vi "Camera Manual Control.vi"() -> ()   [LabVIEW 2017]
uses:
  Shared Components/Gantry Class/Gantry Class.lvclass
  Shared Components/Config Manager Class/Type Definitions/Camera Enum.ctl
panel:
  in  "Enable Crosshairs":bool
  out "error out":errorcluster
  in  "stop":bool
  in  "Camera Name":T1
  out "Preview":T2(plugin-control)
  in  "Virtual Mode":bool
  in  "Config Folder":path=path "C:/Users/husker/Desktop/gantry/Config"
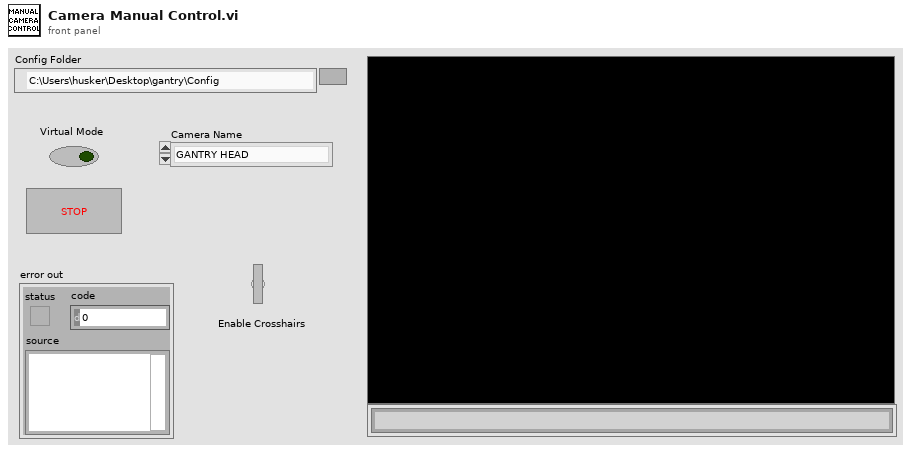
[diagram p1: front panel]
types:
  T1 = typedef "Camera Enum.ctl" = enum16{"GANTRY HEAD", "NEEDLE CALIBRATION X", "NEEDLE CALIBRATION Y", "STAND CAMERA"}
  T2 = typedef "IMAQ Image.ctl" = refnum<image>
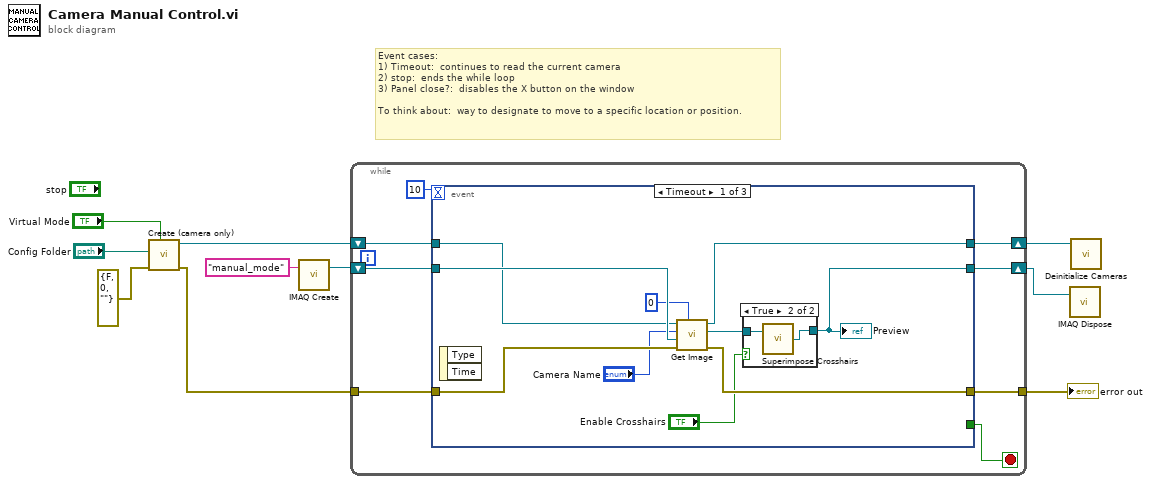
[diagram p0: block diagram]
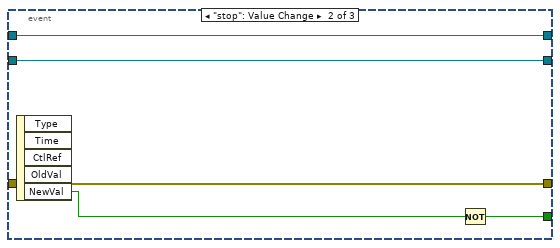
[diagram p3: hidden frame]
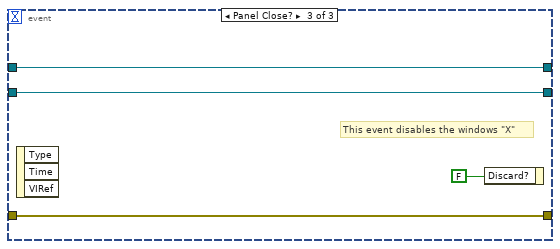
[diagram p4: hidden frame]
diagram:
  # "Event cases:\n1) Timeout:  continues to read the current camera\n2) stop:  ends the while loop\n3) Panel close?:  disables the X button on the window\n\nTo think about:  way to designate to move to a specific location or position."
  n1 = call "Create (camera only).vi"("Virtual Mode"="Virtual Mode", "error in"=errorcluster {"status"=FALSE, "code"=0, "source"=""}, "Config Folder"="Config Folder") -> ("error out"=w4:errorcluster, "Gantry out"=w7:refnum<class "Gantry Class.lvclass">)  [unwired: 7 in]
  n2 = call "IMAQ Create"("Image Name"="manual_mode") -> ("New Image"=w6:T2)  [unwired: 4 in, 1 out]
  n3 = while {
    tunnel: w4 -> [w16]
    tunnel: [w17] -> w2
    shift-right: [w12] -> w1
    shift-left: w6 -> [w13]
    shift-right: [w14] -> w3
    shift-left: w7 -> [w15]
    stop <- w11 stop-if-true
    n4 = event shown="[0] Timeout" {
      selector: _ -> [_ _ _]
      dyn-events: _ -> [_ _ _]
      timeout: 10 -> [_ _ _]
      tunnel: [_ w32 _] -> w11
      tunnel: [w26 w36 w39] -> w17
      tunnel: w16 -> [w23 w36 w39]
      tunnel: w15 -> [w24 w35 w38]
      tunnel: [w28 w35 w38] -> w14
      tunnel: w13 -> [w27 w34 w37]
      tunnel: [w20 w34 w37] -> w12
      event Timeout {
        n5 = event-data() -> ()  [unwired: 1 in, 2 out]
        n6 = call-dynamic "Get Image.vi"("Delay(milliseconds)"=0, "error in"=w23, "Image In"=w27, "Camera Name"="Camera Name", "Gantry in"=w24) -> ("error out"=w26:errorcluster, "Image Out"=w21:T2, "Gantry out"=w28:refnum<class "Gantry Class.lvclass">)  [unwired: 3 in, 1 out]
        n7 = case shown="True" "Enable Crosshairs" {
          tunnel: w21 -> [w29 w31]
          tunnel: [w29 w30] -> w20
          frame False {
          }
          frame True {
            n8 = call "Superimpose Crosshairs.vi"("Refnum in"=w31) -> ("Refnum out"=w30:T2)  [unwired: 1 in]
          }
        }
        "Preview" <- w20
      }
      event "stop": Value Change {
        n9 = event-data() -> ("NewVal"=w33:bool)  [unwired: 1 in, 4 out]
        n10 = Not(x=w33) -> (.not. x?=w32:bool)
      }
      event Panel Close? {
        # "This event disables the windows \"X\""
        n11 = event-data() -> ()  [unwired: 1 in, 3 out]
        n12 = event-data("Discard?"=FALSE) -> ()  [unwired: 1 in, 1 out]
      }
    }
  }
  "error out" <- w2
  n13 = call "IMAQ Dispose"("Image"=w1) -> ()  [unwired: 5 in, 1 out]
  n14 = call-dynamic "Deinitialize Cameras.vi"("Gantry in"=w3) -> ()  [unwired: 9 in, 2 out]
